vi "Emballage_BBD_remplacer_1Valve.vi"(6 "ID_UTILISATEUR_GPAO":string, 8 "Error in":errorcluster caption="Error in (no error)", 9 "No Commande :":string, 10 "Liste Carton":string[](array[string]), 11 "Liste n° pièces de la cmde":string[](array[string])) -> (0 "Error out":errorcluster)   [LabVIEW 2020]
uses:
  Modules/FS/60_FS_Controles/60_FS_SetGet.ctl
panel:
  out "produit scanné_remplacant":string
  in  "remplacer_valve":bool
  in  "Supprimer_valve":bool
  out "SN_Produit :":string
  out "No Carton :":string
  out "indice de l'élément":i32
  out "Annulé/Quitter":bool
  in  "btn_quitter":bool
  # "Information sur le produit scanné:"
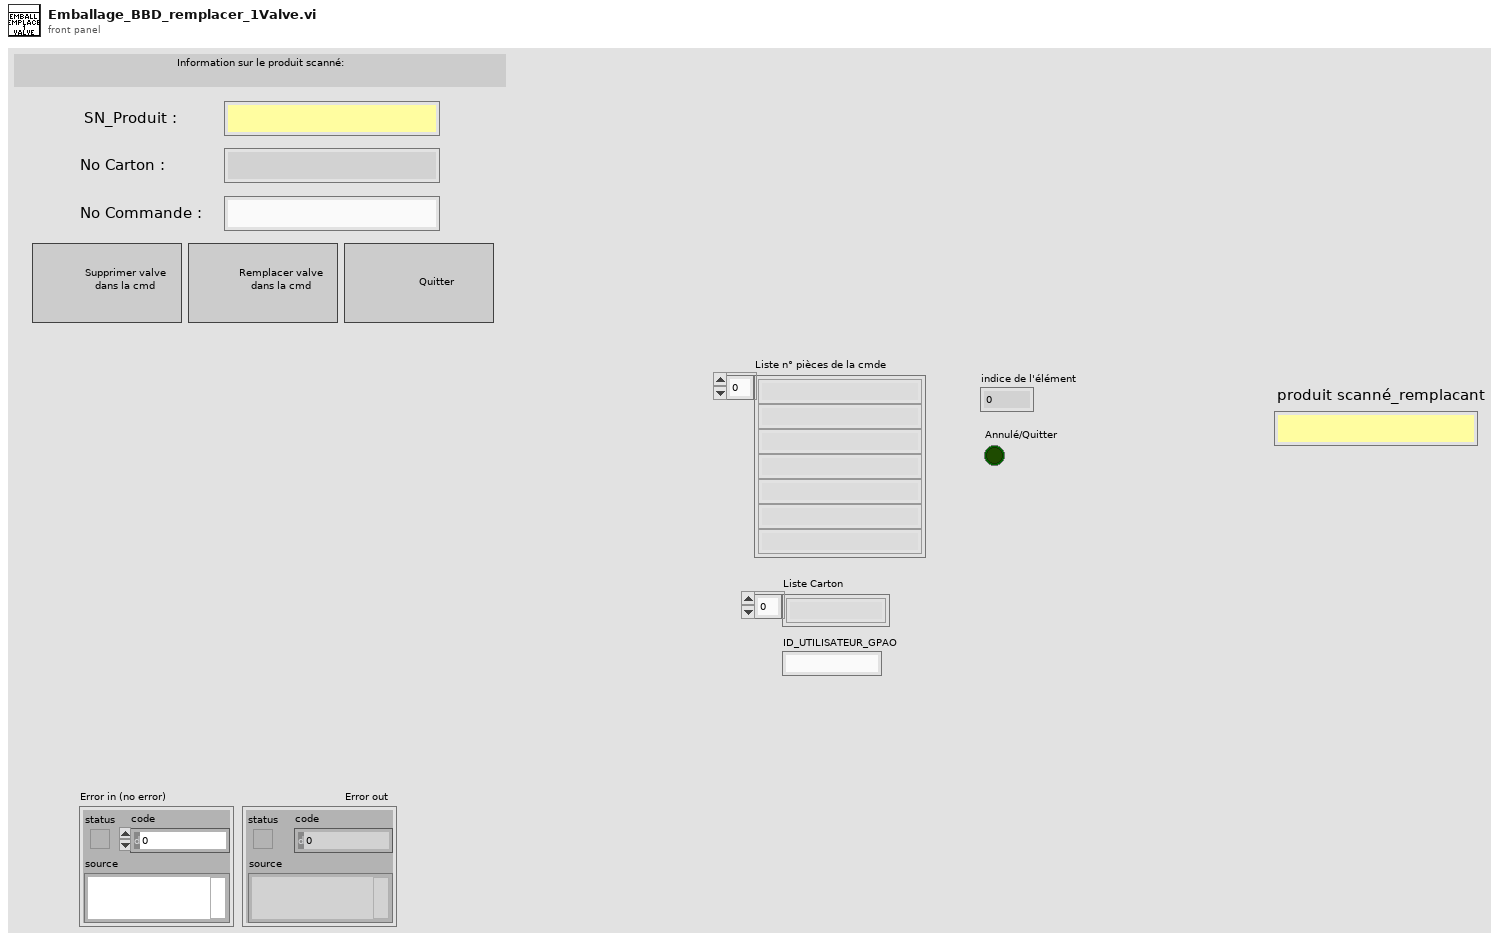
[diagram p1: front panel]
types:
  T1 = typedef "60_FS_SetGet.ctl" = enum16{"set", "get"}
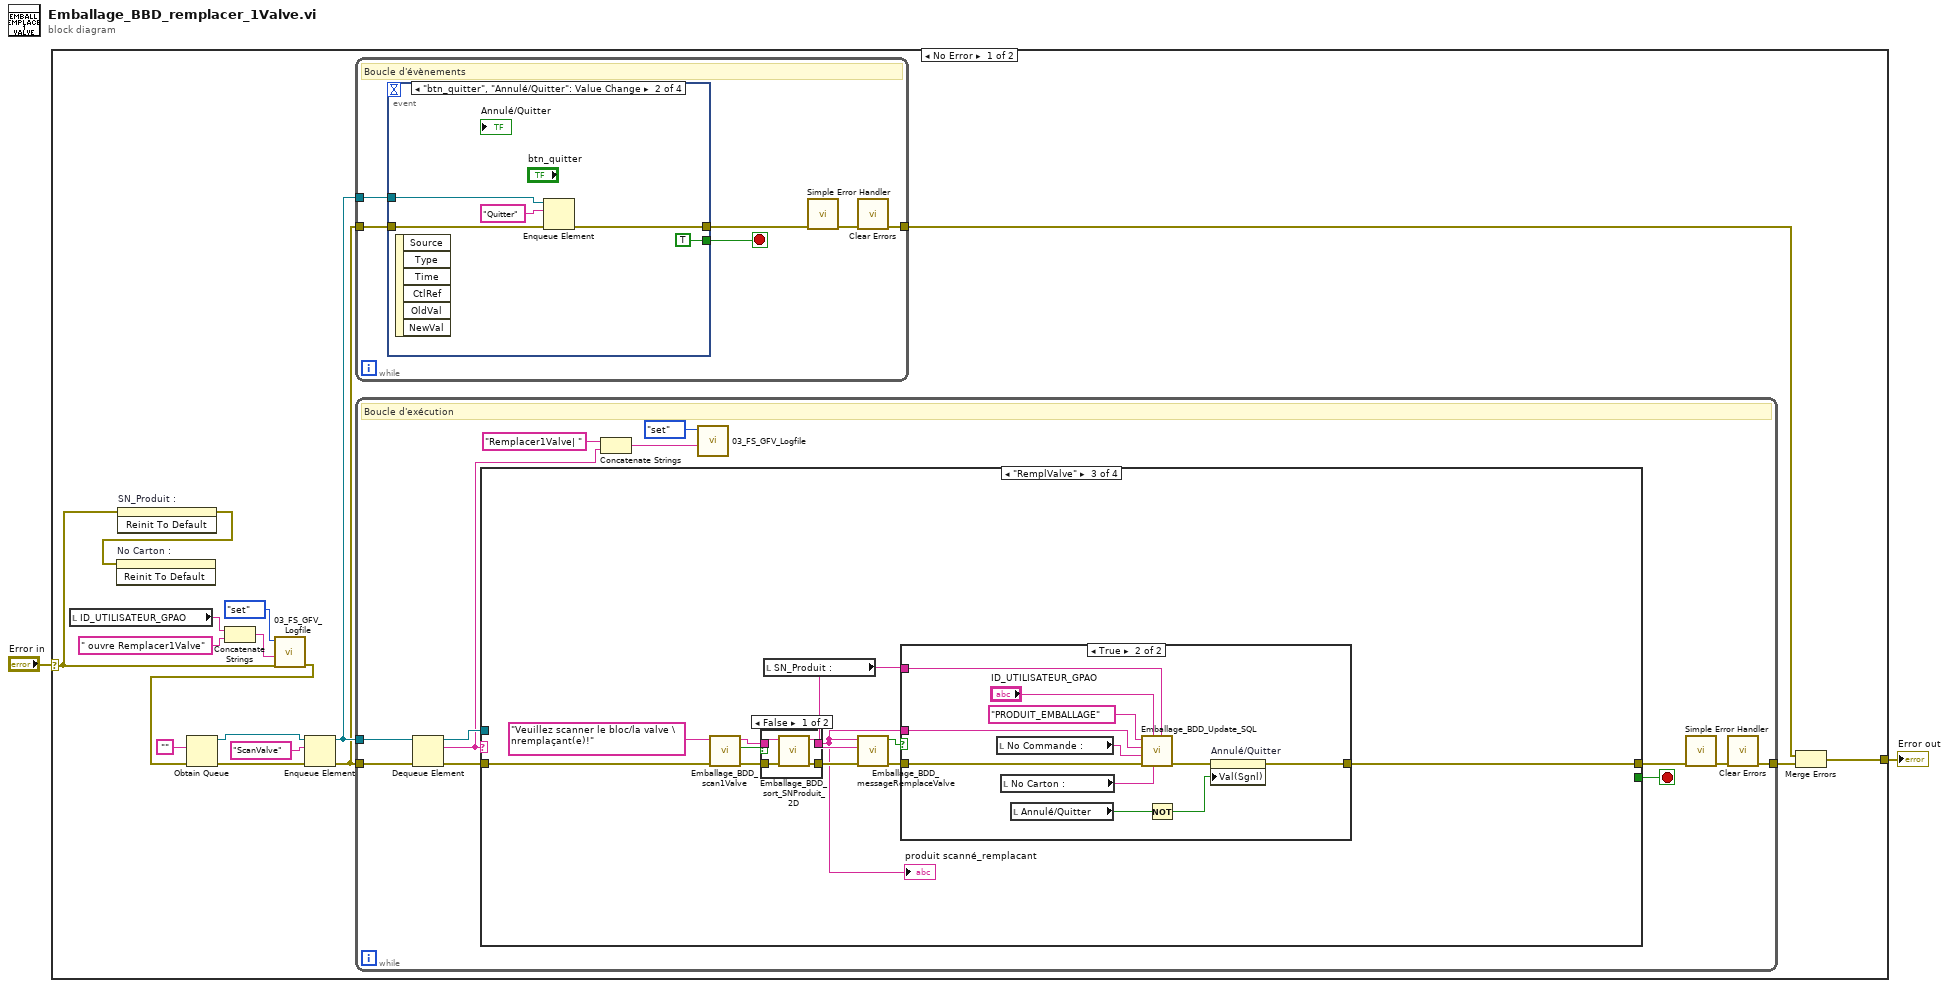
[diagram p0: block diagram]
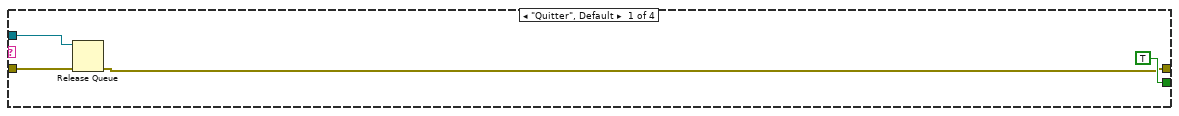
[diagram p2: hidden frame]
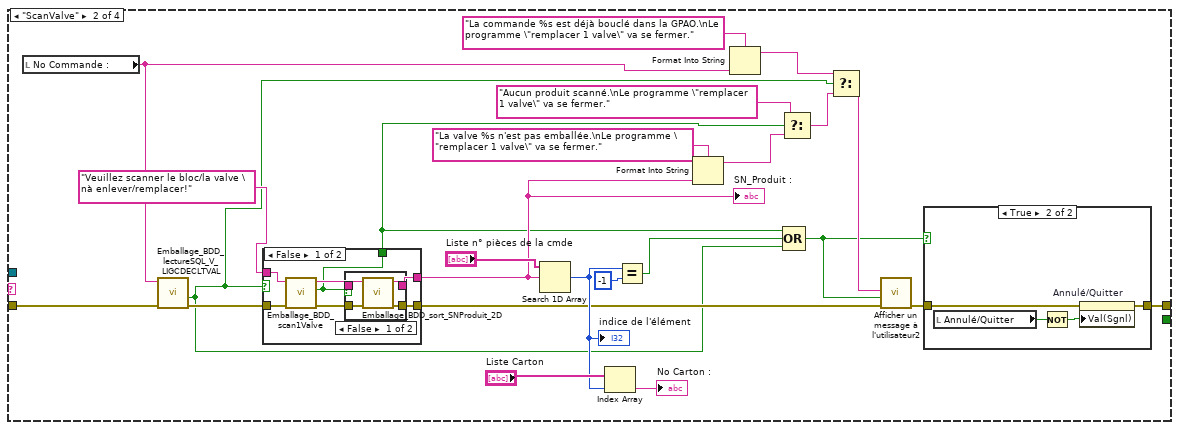
[diagram p3: hidden frame]
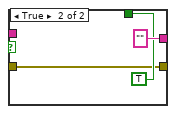
[diagram p5: hidden frame]
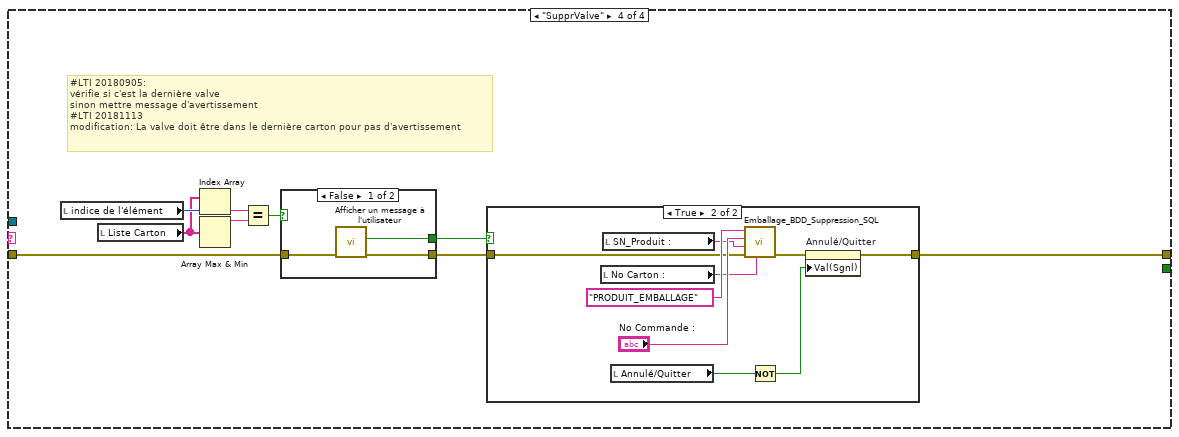
[diagram p9: hidden frame]
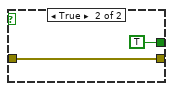
[diagram p10: hidden frame]
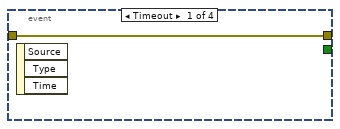
[diagram p12: hidden frame]
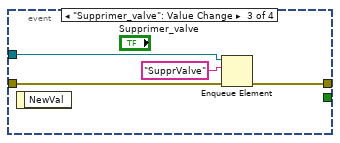
[diagram p13: hidden frame]
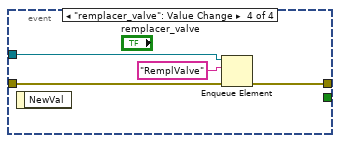
[diagram p14: hidden frame]
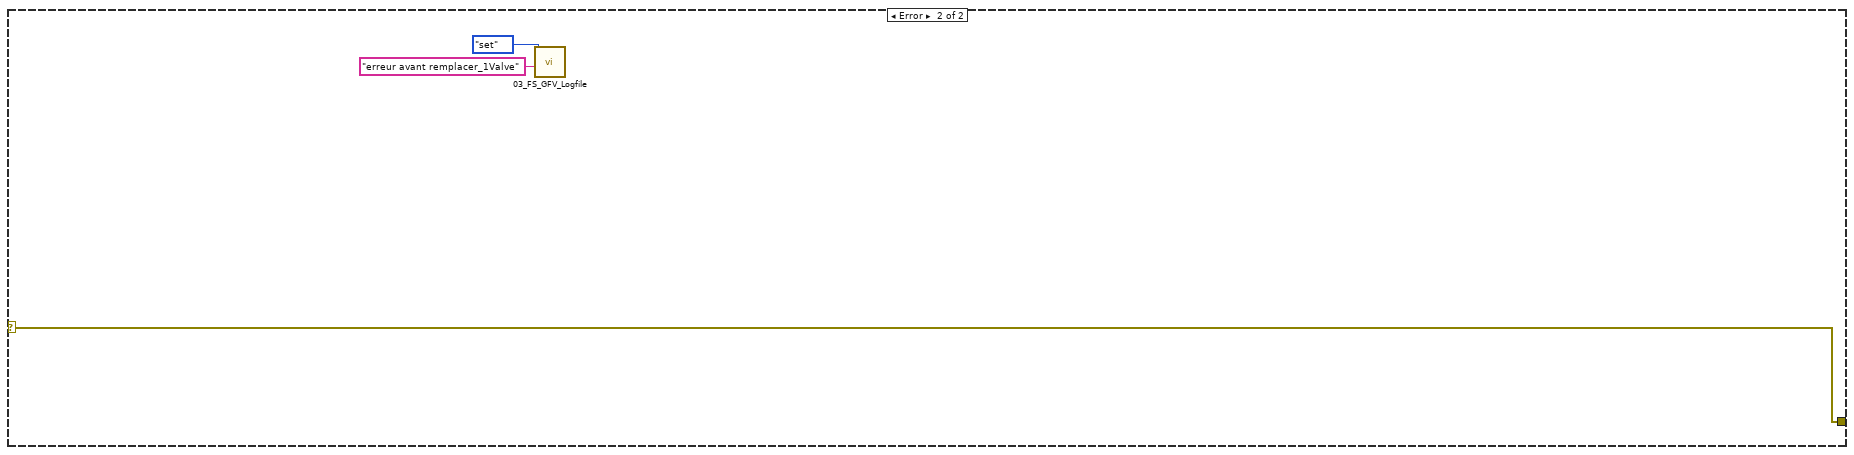
[diagram p15: hidden frame]
diagram:
  n1 = case shown="No Error" "Error in" {
    selector: "Error in" -> [w3 w155]
    tunnel: [w5 w155] -> w1
    frame No Error {
      n2 = local read "ID_UTILISATEUR_GPAO"() -> (w6:string)
      n3 = invoke on="SN_Produit :" class="Ch" method="Reinit To Default"(error in=w3) -> (error out=w4:errorcluster)  [unwired: 2 in, 2 out]
      n4 = invoke on="No Carton :" class="Ch" method="Reinit To Default"(error in=w4) -> ()  [unwired: 2 in, 3 out]
      n5 = Concatenate Strings(w6, " ouvre Remplacer1Valve" ("chaîne")) -> (w8:string)
      n6 = call "03_FS_GFV_Logfile.vi"("error in"=w3, "Chaîne"=w8, "States"=60_FS_SetGet."set") -> ("error out"=w9:errorcluster)  [unwired: 7 in, 1 out]
      n7 = Obtain Queue(element data type="", error in (no error)=w9) -> (queue out=w14:refnum<queue>, error out=w15:errorcluster)  [unwired: 3 in, 1 out]
      n8 = Enqueue Element(queue=w14, element="ScanValve" ("élément"), error in (no error)=w15) -> (queue out=w12:refnum<queue>, error out=w11:errorcluster)  [unwired: 1 in, 1 out]
      n9 = while {
        tunnel: [w138] -> w17
        tunnel: w12 -> [w135]
        tunnel: w11 -> [w134]
        stop <- w136 stop-if-true
        # "Boucle d'évènements"
        n10 = event shown="[1] \"btn_quitter\", \"Annulé/Quitter\": Value Change" {
          selector: _ -> [_ _ _ _]
          dyn-events: _ -> [_ _ _ _]
          timeout: _ -> [_ _ _ _]
          tunnel: [_ TRUE _ _] -> w136
          tunnel: w135 -> [_ w143 w146 w150]
          tunnel: w134 -> [w139 w142 w148 w152]
          tunnel: [w139 w140 w147 w151] -> w133
          event Timeout {
            n11 = event-data() -> ()  [unwired: 1 in, 3 out]
          }
          event "btn_quitter", "Annulé/Quitter": Value Change {
            n12 = event-data() -> ()  [unwired: 1 in, 6 out]
            n13 = Enqueue Element(queue=w143, element="Quitter" ("élément"), error in (no error)=w142) -> (error out=w140:errorcluster)  [unwired: 1 in, 2 out]
          }
          event "Supprimer_valve": Value Change {
            n14 = event-data() -> ()  [unwired: 1 in, 1 out]
            n15 = Enqueue Element(queue=w146, element="SupprValve" ("élément"), error in (no error)=w148) -> (error out=w147:errorcluster)  [unwired: 1 in, 2 out]
          }
          event "remplacer_valve": Value Change {
            n16 = event-data() -> ()  [unwired: 1 in, 1 out]
            n17 = Enqueue Element(queue=w150, element="RemplValve" ("élément"), error in (no error)=w152) -> (error out=w151:errorcluster)  [unwired: 1 in, 2 out]
          }
        }
        n18 = call <vilib>:"Simple Error Handler.vi"("error in (no error)"=w133) -> ("error out"=w137:errorcluster)  [unwired: 4 in, 4 out]
        n19 = call <vilib>:"Clear Errors.vi"("error in (no error)"=w137) -> ("error out"=w138:errorcluster)  [unwired: 5 in, 1 out]
      }
      n20 = while {
        tunnel: w12 -> [w30]
        tunnel: [w28] -> w16
        tunnel: w11 -> [w26]
        stop <- w25 stop-if-true
        # "Boucle d'exécution"
        n21 = Dequeue Element(queue=w30, error in (no error)=w26) -> (queue out=w24:refnum<queue>, element=w20:string, error out=w23:errorcluster)  [unwired: 1 in, 1 out]
        n22 = case shown="\"RemplValve\"" w20 {
          tunnel: [TRUE _ _ _] -> w25
          tunnel: w24 -> [w33 _ _ _]
          tunnel: w23 -> [w32 w43 w90 w114]
          tunnel: [w31 w50 w88 w117] -> w22
          frame "Quitter", Default {
            n23 = Release Queue(queue=w33, error in (no error)=w32) -> (error out=w31:errorcluster)  [unwired: 1 in, 2 out]
          }
          frame "ScanValve" {
            n24 = local read "No Commande :"() -> (w45:string)
            n25 = call "Emballage_BDD_lectureSQL_V_LIGCDECLTVAL.vi"("Error in"=w43, "NO_CDEVAL"=w45) -> ("Error out"=w42:errorcluster, "CMD_DejaBoucle?"=w40:bool)  [unwired: 6 in, 2 out]
            n26 = case shown="False" w40 {
              tunnel: [w59 TRUE ("Annulé?")] -> w38
              tunnel: "Veuillez scanner le bloc/la valve \nà enlever/remplacer!" ("Instruction_IN") -> [w65 _]
              tunnel: [w60 "" ("produit scanné:")] -> w53
              tunnel: w42 -> [w64 w72]
              tunnel: [w62 w72] -> w41
              frame False {
                n27 = call "Emballage_BDD_scan1Valve.vi"("Error in"=w64, "Instruction_IN"=w65) -> ("Error out"=w63:errorcluster, "TIMEOUT_FIN?"=w59:bool, "produit scanné:"=w61:string)  [unwired: 7 in]
                n28 = case shown="False" w59 {
                  tunnel: w63 -> [w69 w71]
                  tunnel: [w68 w71] -> w62
                  tunnel: w61 -> [w67 w70]
                  tunnel: [w66 w70] -> w60
                  frame False {
                    n29 = call "Emballage_BDD_sort_SNProduit_2D.vi"("Error in"=w69, "Chaine_Lecteur"=w67) -> ("Error out"=w68:errorcluster, "SN_PRODUIT"=w66:string)  [unwired: 4 in, 4 out]
                  }
                  frame True {
                  }
                }
              }
              frame True {
              }
            }
            "SN_Produit :" <- w53
            n30 = Search 1D Array(1D array="Liste n° pièces de la cmde", element=w53) -> (index of element=w52:i32)  [unwired: 1 in]
            "indice de l'élément" <- w52
            n31 = Index Array(array="Liste Carton", index=w52) -> (element=→"No Carton :":string)
            n32 = Equal?(x=w52, y=-1) -> (x = y?=w48:bool)
            n33 = Format Into String(format string="La valve %s n'est pas emballée.\nLe programme \"remplacer 1 valve\" va se fermer." ("Message"), w53) -> (resulting string=w37:string)  [unwired: 2 in, 1 out]
            n34 = Format Into String(format string="La commande %s est déjà bouclé dans la GPAO.\nLe programme \"remplacer 1 valve\" va se fermer." ("Message"), w45) -> (resulting string=w46:string)  [unwired: 2 in, 1 out]
            n35 = Select(t="Aucun produit scanné.\nLe programme \"remplacer 1 valve\" va se fermer." ("Message"), s=w38, f=w37) -> (s? t:f=w39:string)
            n36 = Compound Arithmetic op=OR ("Opérateur arithmétique")(w38, w48, w40) -> (w35:bool)
            n37 = Select(t=w46, s=w40, f=w39) -> (s? t:f=w47:string)
            n38 = call "Afficher un message à l'utilisateur2"("error in (no error)"=w41, "Enable"=w35, "Message"=w47) -> ("error out"=w49:errorcluster)  [unwired: 7 in, 1 out]
            n39 = case shown="True" w35 {
              tunnel: w49 -> [w75 w77]
              tunnel: [w75 w76] -> w50
              frame False {
              }
              frame True {
                n40 = local read "Annulé/Quitter"() -> (w79:bool)
                n41 = Not(x=w79) -> (.not. x?=w78:bool)
                n42 = property on="Annulé/Quitter" class="Bool (strict)"(error in=w77, "Val(Sgnl)"=w78) -> (error out=w76:errorcluster)  [unwired: 1 in, 1 out]
              }
            }
          }
          frame "RemplValve" {
            n43 = call "Emballage_BDD_scan1Valve.vi"("Error in"=w90, "Instruction_IN"="Veuillez scanner le bloc/la valve \nremplaçant(e)!") -> ("Error out"=w83:errorcluster, "TIMEOUT_FIN?"=w80:bool, "produit scanné:"=w82:string)  [unwired: 7 in]
            n44 = case shown="False" w80 {
              tunnel: w83 -> [w94 w96]
              tunnel: [w93 w96] -> w84
              tunnel: w82 -> [w92 w95]
              tunnel: [w91 w95] -> w81
              frame False {
                n45 = call "Emballage_BDD_sort_SNProduit_2D.vi"("Error in"=w94, "Chaine_Lecteur"=w92) -> ("Error out"=w93:errorcluster, "SN_PRODUIT"=w91:string)  [unwired: 4 in, 4 out]
              }
              frame True {
              }
            }
            "produit scanné_remplacant" <- w81
            n46 = local read "SN_Produit :"() -> (w86:string)
            n47 = call "Emballage_BDD_messageRemplaceValve.vi"("Error in"=w84, "SN_RPODUIT_ancien"=w86, "SN_PRODUIT remplacant"=w81) -> ("Error out"=w87:errorcluster, "btn_Continuer 2"=w85:bool)  [unwired: 7 in]
            n48 = case shown="True" w85 {
              tunnel: [w97 w101] -> w88
              tunnel: w81 -> [_ w105]
              tunnel: w87 -> [w97 w104]
              tunnel: w86 -> [_ w103]
              frame False {
              }
              frame True {
                n49 = local read "No Commande :"() -> (w106:string)
                n50 = local read "No Carton :"() -> (w107:string)
                n51 = local read "Annulé/Quitter"() -> (w100:bool)
                n52 = call "Emballage_BDD_Update_SQL.vi"("SN_PRODUIT ancien"=w103, "NO_DU_CARTON"=w107, "ID_UTILISATEUR_GPAO"="ID_UTILISATEUR_GPAO", "error in (no error)"=w104, "NO_CDEVAL"=w106, "SN_PRODUIT"=w105, "Table"="PRODUIT_EMBALLAGE") -> ("error out"=w102:errorcluster)  [unwired: 4 in]
                n53 = Not(x=w100) -> (.not. x?=w99:bool)
                n54 = property on="Annulé/Quitter" class="Bool (strict)"(error in=w102, "Val(Sgnl)"=w99) -> (error out=w101:errorcluster)  [unwired: 1 in, 1 out]
              }
            }
          }
          frame "SupprValve" {
            # "#LTI 20180905:\nvérifie si c'est la dernière valve\nsinon mettre message d'avertissement\n#LTI 20181113\nmodification: La valve doit être dans le dernière carton pour pas d'avertissement"
            n55 = local read "indice de l'élément"() -> (w112:i32)
            n56 = local read "Liste Carton"() -> (w110:string[])
            n57 = Index Array(array=w110, index=w112) -> (element=w111:string)
            n58 = Array Max & Min(array=w110) -> (max value=w109:string)  [unwired: 3 out]
            n59 = Equal?(x=w111, y=w109) -> (x = y?=w116:bool)
            n60 = case shown="False" w116 {
              tunnel: [w118 TRUE] -> w115
              tunnel: w114 -> [w120 w121]
              tunnel: [w119 w121] -> w113
              frame False {
                n61 = call "Afficher un message à l'utilisateur"("error in (no error)"=w120) -> ("error out"=w119:errorcluster, "Oui, supprimer valve"=w118:bool)  [unwired: 9 in]
              }
              frame True {
              }
            }
            n62 = case shown="True" w115 {
              tunnel: w113 -> [w123 w129]
              tunnel: [w123 w124] -> w117
              frame False {
              }
              frame True {
                n63 = local read "No Carton :"() -> (w128:string)
                n64 = local read "SN_Produit :"() -> (w130:string)
                n65 = local read "Annulé/Quitter"() -> (w127:bool)
                n66 = call "Emballage_BDD_Suppression_SQL.vi"("NO_DU_CARTON"=w128, "error in (no error)"=w129, "SN_PRODUIT"=w130, "NO_CDEVAL"="No Commande :", "Table"="PRODUIT_EMBALLAGE") -> ("error out"=w125:errorcluster)  [unwired: 6 in]
                n67 = Not(x=w127) -> (.not. x?=w126:bool)
                n68 = property on="Annulé/Quitter" class="Bool (strict)"(error in=w125, "Val(Sgnl)"=w126) -> (error out=w124:errorcluster)  [unwired: 1 in, 1 out]
              }
            }
          }
        }
        n69 = Concatenate Strings("Remplacer1Valve| " ("chaîne"), w20) -> (w21:string)
        n70 = call "03_FS_GFV_Logfile.vi"("Chaîne"=w21, "States"=60_FS_SetGet."set") -> ()  [unwired: 8 in, 2 out]
        n71 = call <vilib>:"Simple Error Handler.vi"("error in (no error)"=w22) -> ("error out"=w27:errorcluster)  [unwired: 4 in, 4 out]
        n72 = call <vilib>:"Clear Errors.vi"("error in (no error)"=w27) -> ("error out"=w28:errorcluster)  [unwired: 5 in, 1 out]
      }
      n73 = Merge Errors(w17, w16) -> (w5:errorcluster)
    }
    frame Error {
      n74 = call "03_FS_GFV_Logfile.vi"("Chaîne"="erreur avant remplacer_1Valve", "States"=60_FS_SetGet."set") -> ()  [unwired: 8 in, 2 out]
    }
  }
  "Error out" <- w1
